vi "CfgManager.Collection Test Launcher.vi"() -> ()   [LabVIEW 2013]
uses:
  <vilib>/LabVIEW Open Source Project/Unicity/Delimiter/Delimiters List.ctl
  Manager.Text/ConfigManager.Text.lvclass
  Manager.Text/ConfigManager.Text.lvclass/ConfigManager.Text.ctl
  Collection/ConfigManagerCollection.lvclass
  Manager/Decompose KVPs.vi
  Manager/Write.vi
  Manager/Read.vi
  <vilib>/LabVIEW Open Source/Data Manipulation/KVP Parser.vi
  Manager/ConfigManager.lvclass
  Cache/ConfigManager.Cache.lvclass
  <vilib>/LabVIEW Open Source Project/Unicity/Delimiter/Delimiter.lvclass
panel:
  out "modified PID settings":variant
  out "all found? 3":bool
  out "all found? 2":bool
  out "all found?":bool
  out "user-defined pump config":variant
  out "default pump config":variant
  in  "default config":path
  out "merged PID settings":variant
  out "initial PID settings":variant
  out "System.Valve Keys":string[](array[string])
  out "System.Pump keys":string[](array[string])
  out "modified pump config":variant
  out "error out":errorcluster
  out "merged pump config":variant
  in  "user-defined config":path
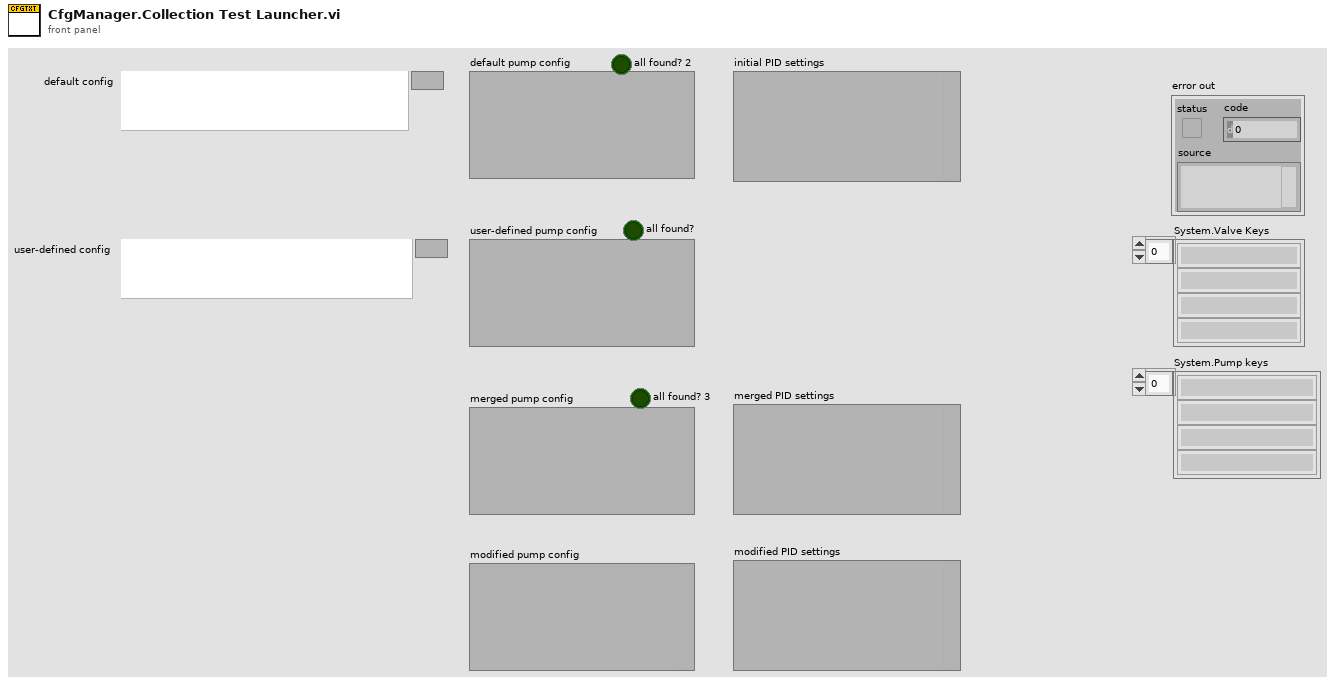
[diagram p1: front panel]
types:
  T1 = cluster{"String":string, "Numeric":dbl, "Boolean":bool}
  T2 = typedef "Delimiter.lvclass/Delimiters List.ctl" = enum16{"Default", "dot (.)", "colon (:)", "double-colon (::)", "semi-colon (;)", "underscore (_)", "double underscore (__)", "dash (-)", "double dash (--)", "backslash (\\)", "vertical bar (|)", "forward slash (/)", "chevron (>)", "double-chevron (>>)", "arrow (->)", "comma (,)", "arobas (@)", "ampersand (&)", "other"}
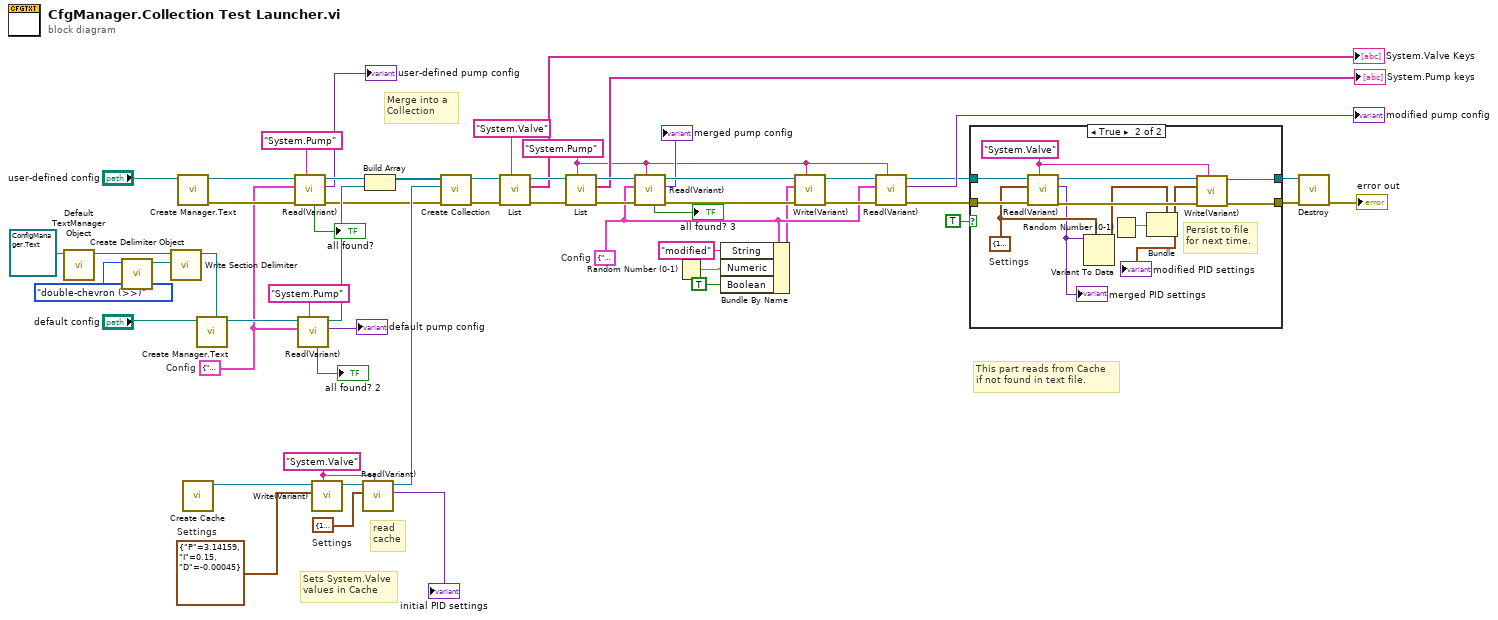
[diagram p0: block diagram]
diagram:
  w5 = T1 {"String"="", "Numeric"=0.0, "Boolean"=FALSE}  # Config
  w21 = cluster{"P":dbl, "I":dbl, "D":dbl} {"P"=1.0, "I"=0.0, "D"=0.0}  # Settings
  w37 = cluster{"P":dbl, "I":dbl, "D":dbl} {"P"=3.14159, "I"=0.15, "D"=-0.00045}  # Settings
  w22 = "System.Valve" ("Qualified Name")
  w39 = "System.Pump" ("Qualified Name")
  w38 = T1 {"String"="", "Numeric"=0.0, "Boolean"=FALSE}  # Config
  # "read\ncache"
  # "This part reads from Cache\nif not found in text file."
  # "Merge into a \nCollection"
  # "Sets System.Valve\nvalues in Cache"
  n1 = call-dynamic "Default TextManager Object.vi"("CfgManager.Text in"=refnum<class "ConfigManager.Text.lvclass"> refnum) -> ("CfgManager.Text out"=w17:refnum<class "ConfigManager.Text.lvclass">)  [unwired: 10 in]
  n2 = call <vilib>:"Create Delimiter Object.vi"("Delimiter"=Delimiters_List."double-chevron (>>)") -> ("Delimiter"=w18:refnum<class "Delimiter.lvclass">)  [unwired: 10 in]
  n3 = call "Write Section Delimiter.vi"("Section Delimiter"=w18, "ConfigManager.Text in"=w17) -> ("ConfigManager.Text out"=w16:refnum<class "ConfigManager.Text.lvclass">)  [unwired: 9 in]
  n4 = call "Create Manager.Text.vi"("filepath"="user-defined config") -> ("error out"=w10:errorcluster, "ConfigManager.Text out"=w8:refnum<class "ConfigManager.Text.lvclass">)  [unwired: 8 in, 1 out]
  n5 = call "Create Cache.vi"() -> ("ConfigManager.Cache"=w36:refnum<class "ConfigManager.Cache.lvclass">)  [unwired: 11 in]
  n6 = call "Create Manager.Text.vi"("ConfigManager.Text"=w16, "filepath"="default config") -> ("ConfigManager.Text out"=w14:refnum<class "ConfigManager.Text.lvclass">)  [unwired: 7 in, 2 out]
  n7 = call "Read(Variant).vi"("Qualified Name"="System.Pump", "error in (no error)"=w10, "Type"=w5, "ConfigManager in"=w8) -> ("error out"=w9:errorcluster, "value"=→"user-defined pump config":variant, "ConfigManager out"=w7:refnum<class "ConfigManager.Text.lvclass">, "all found?"=→"all found?":bool)  [unwired: 3 in, 1 out]
  n8 = call "Read(Variant).vi"("Qualified Name"="System.Pump", "Type"=w5, "ConfigManager in"=w14) -> ("value"=→"default pump config":variant, "ConfigManager out"=w13:refnum<class "ConfigManager.Text.lvclass">, "all found?"=→"all found? 2":bool)  [unwired: 4 in, 2 out]
  n9 = call "Write(Variant).vi"("Qualified Name"=w22, "value"=w37, "ConfigManager in"=w36) -> ("ConfigManager out"=w25:refnum<class "ConfigManager.Cache.lvclass">)  [unwired: 6 in, 2 out]
  n10 = call "Read(Variant).vi"("Qualified Name"=w22, "Type"=w21, "ConfigManager in"=w25) -> ("value"=→"initial PID settings":variant, "ConfigManager out"=w24:refnum<class "ConfigManager.Cache.lvclass">)  [unwired: 4 in, 3 out]
  n11 = Build Array(w7, w13) -> (w26:refnum<class "ConfigManager.Text.lvclass">[])
  n12 = call "Create Collection.vi"("Cache"=w24, "List"=w26) -> ("ConfigManagerCollection out"=w35:refnum<class "ConfigManagerCollection.lvclass">)  [unwired: 9 in]
  n13 = call "List.vi"("Qualified Name"="System.Valve", "error in (no error)"=w9, "ConfigManager in"=w35) -> ("error out"=w33:errorcluster, "Keys"=→"System.Valve Keys":string[], "ConfigManager out"=w34:refnum<class "ConfigManagerCollection.lvclass">)  [unwired: 6 in]
  n14 = call "List.vi"("Qualified Name"=w39, "error in (no error)"=w33, "ConfigManager in"=w34) -> ("error out"=w48:errorcluster, "Keys"=→"System.Pump keys":string[], "ConfigManager out"=w47:refnum<class "ConfigManagerCollection.lvclass">)  [unwired: 6 in]
  n15 = call "Read(Variant).vi"("Qualified Name"=w39, "error in (no error)"=w48, "Type"=w38, "ConfigManager in"=w47) -> ("error out"=w52:errorcluster, "value"=→"merged pump config":variant, "ConfigManager out"=w53:refnum<class "ConfigManagerCollection.lvclass">, "all found?"=→"all found? 3":bool)  [unwired: 3 in, 1 out]
  n16 = Random Number (0-1)() -> (number: 0 to 1=w28:dbl)
  n17 = Bundle By Name(cluster=w38, "String"="modified", "Numeric"=w28, "Boolean"=TRUE) -> (w27:T1)
  n18 = call "Write(Variant).vi"("Qualified Name"=w39, "error in (no error)"=w52, "value"=w27, "ConfigManager in"=w53) -> ("error out"=w50:errorcluster, "ConfigManager out"=w51:refnum<class "ConfigManagerCollection.lvclass">)  [unwired: 5 in, 1 out]
  n19 = call "Read(Variant).vi"("Qualified Name"=w39, "error in (no error)"=w50, "Type"=w38, "ConfigManager in"=w51) -> ("error out"=w42:errorcluster, "value"=→"modified pump config":variant, "ConfigManager out"=w44:refnum<class "ConfigManagerCollection.lvclass">)  [unwired: 3 in, 2 out]
  n20 = case shown="True" TRUE {
    tunnel: w44 -> [w57 w69]
    tunnel: [w57 w64] -> w43
    tunnel: w42 -> [w56 w68]
    tunnel: [w56 w63] -> w41
    frame False {
    }
    frame True {
      w62 = cluster{"P":dbl, "I":dbl, "D":dbl} {"P"=1.0, "I"=0.0, "D"=0.0}  # Settings
      w65 = "System.Valve" ("Qualified Name")
      # "Persist to file\nfor next time."
      n21 = call "Read(Variant).vi"("Qualified Name"=w65, "error in (no error)"=w68, "Type"=w62, "ConfigManager in"=w69) -> ("error out"=w66:errorcluster, "value"=w61:variant, "ConfigManager out"=w67:refnum<class "ConfigManagerCollection.lvclass">)  [unwired: 3 in, 2 out]
      "merged PID settings" <- w61
      n22 = Variant To Data(type=w62, Variant=w61) -> (data=w59:cluster{"P":dbl, "I":dbl, "D":dbl})  [unwired: 1 in, 1 out]
      n23 = Random Number (0-1)() -> (number: 0 to 1=w60:dbl)
      n24 = Bundle(cluster=w59, "I"=w60) -> (w58:cluster{"P":dbl, "I":dbl, "D":dbl})  [unwired: 2 in]
      "modified PID settings" <- w58
      n25 = call "Write(Variant).vi"("Qualified Name"=w65, "error in (no error)"=w66, "value"=w58, "ConfigManager in"=w67) -> ("error out"=w63:errorcluster, "ConfigManager out"=w64:refnum<class "ConfigManagerCollection.lvclass">)  [unwired: 5 in, 1 out]
    }
  }
  n26 = call-dynamic "Destroy.vi"("error in (no error)"=w41, "ConfigManagerCollection in"=w43) -> ("error out"=→"error out":errorcluster)  [unwired: 8 in, 1 out]
